vi "InAs TED Characterise - VoltageInput plus temperature.vi"() -> ()   [LabVIEW 2024]
uses:
  <instrlib>/Keithley DMM6500 DAQ6500 Series/Public/Data/Read (Single Point).vi
  <instrlib>/Keithley DMM6500 DAQ6500 Series/Keithley DMM6500 DAQ6500 Series.lvlib
panel:
  in  "Avg Count":u32=10
  in  "stop":bool
  out "element":dbl
  in  "Tab Control":enum32{"Page 1", "Page 2"}(tab)
  out "InAs Detector Response":cluster{dbl[], dbl[]}[](graph)
  out "Temperature Chart":dynamicdata(graph)
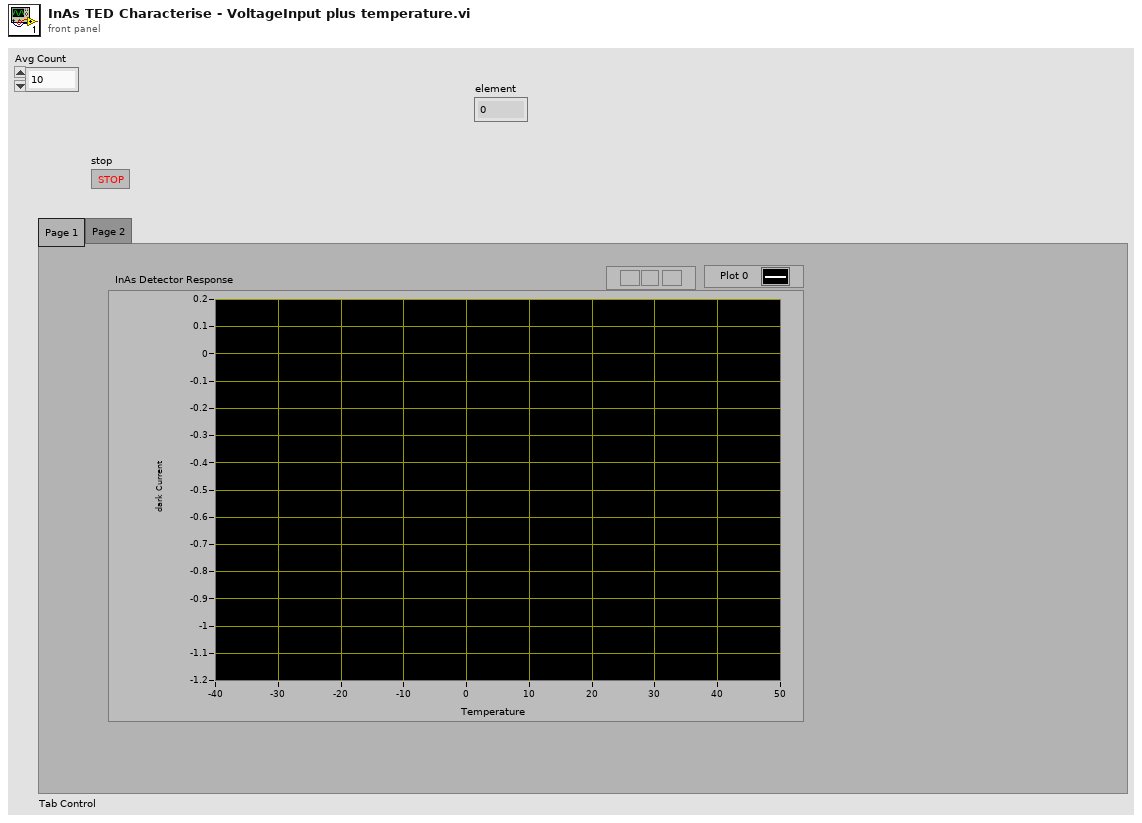
[diagram p1: front panel]
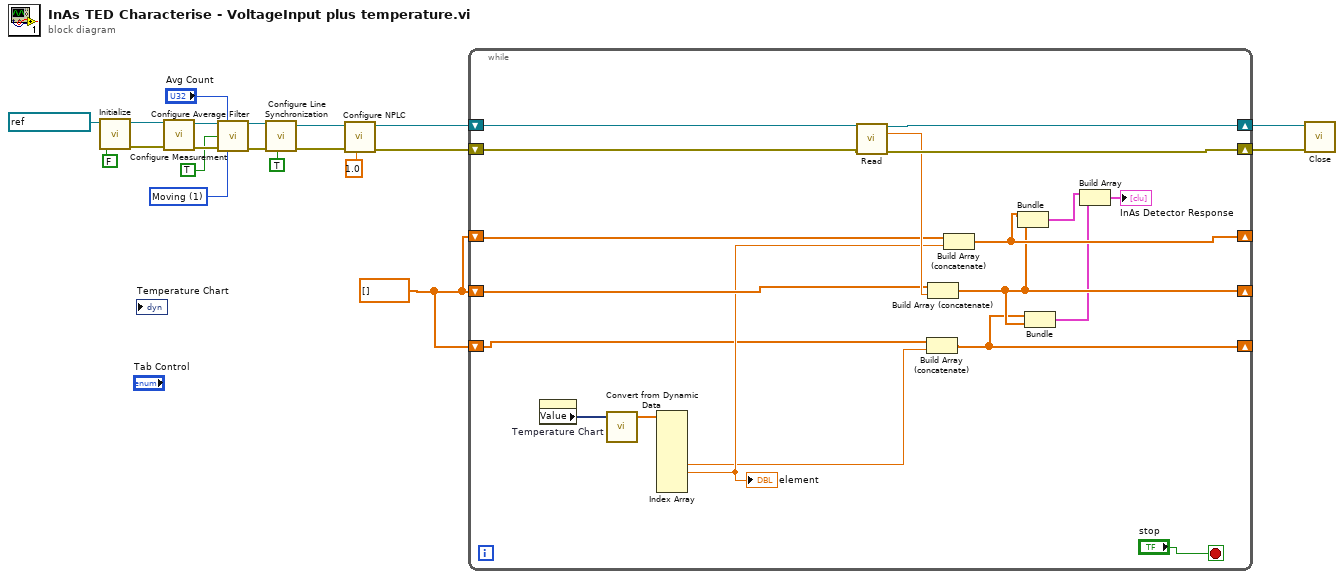
[diagram p0: block diagram]
diagram:
  w10 = 1 items=["Repeat", "Moving"] ("Average Filter Type (0: Repeat)")
  w1 = dbl[] []
  n1 = call <instrlib>:"Initialize.vi"("ID Query (True)"=FALSE ("Reset (True)"), "VISA resource name"=refnum<visa-resource-name> "DMM6500") -> ("error out"=w11:errorcluster, "VISA resource name out"=w12:refnum<visa-resource-name>)  [unwired: 8 in]
  n2 = call <instrlib>:"Configure Measurement.vi"("error in (no error)"=w11, "VISA resource name"=w12) -> ("error out"=w15:errorcluster, "VISA resource name out"=w16:refnum<visa-resource-name>)  [unwired: 8 in]
  n3 = call <instrlib>:"Configure Average Filter.vi"("VISA resource name"=w16, "Count (10)"="Avg Count", "Enable Average Filter (F: Disable)"=TRUE, "error in (no error)"=w15, "Average Filter Type (0: Repeat)"=w10) -> ("VISA resource name out"=w8:refnum<visa-resource-name>, "error out"=w9:errorcluster)  [unwired: 9 in]
  n4 = call <instrlib>:"Configure Line Synchronization.vi"("Enable Line Sync (F: Disable)"=TRUE, "error in (no error)"=w9, "VISA resource name"=w8) -> ("error out"=w6:errorcluster, "VISA resource name out"=w5:refnum<visa-resource-name>)  [unwired: 7 in]
  n5 = call <instrlib>:"Configure NPLC.vi"("Power Line Cycle (1)"=1.0, "error in (no error)"=w6, "VISA resource name"=w5) -> ("error out"=w3:errorcluster, "VISA resource name out"=w4:refnum<visa-resource-name>)  [unwired: 7 in]
  n6 = while {
    shift-right: [w39] -> w19
    shift-left: w4 -> [w37]
    shift-right: [w38] -> w18
    shift-left: w3 -> [w36]
    shift-right: [w25] -> _
    shift-left: w1 -> [w32]
    shift-right: [w29] -> _
    shift-left: w1 -> [w31]
    shift-right: [w24] -> _
    shift-left: w1 -> [w27]
    stop <- "stop" stop-if-true
    n7 = property on="Temperature Chart" class="WFChart (strict)"() -> ("Value"=w34:dynamicdata)  [unwired: 2 in, 2 out]
    n8 = call "Convert from Dynamic Data"("Dynamic Data Type"=w34) -> ("Array"=w33:dbl[])  [unwired: 3 in]
    n9 = Index Array(array=w33) -> (element #5=w26:dbl, element #6=w28:dbl)  [unwired: 8 in, 6 out]
    "element" <- w28
    n10 = call-poly <instrlib>:"Read.vi"("VISA resource name"=w37, "error in (no error)"=w36) -> ("VISA resource name out"=w39:refnum<visa-resource-name>, "Measurement"=w35:dbl, "error out"=w38:errorcluster)  [unwired: 11 in]
    n11 = Build Array (concatenate)(w27, w26) -> (w24:dbl[])
    n12 = Build Array (concatenate)(w32, w35) -> (w25:dbl[])
    n13 = Build Array (concatenate)(w31, w28) -> (w29:dbl[])
    n14 = Bundle(w29, w25) -> (w23:cluster{dbl[], dbl[]})  [unwired: 1 in]
    n15 = Bundle(w24, w25) -> (w22:cluster{dbl[], dbl[]})  [unwired: 1 in]
    n16 = Build Array(w23, w22) -> (→"InAs Detector Response":cluster{dbl[], dbl[]}[])
  }
  n17 = call <instrlib>:"Close.vi"("error in (no error)"=w18, "VISA resource name"=w19) -> ()  [unwired: 9 in, 1 out]
